vi "chooseParametersFromFiles.vi"(0 "Game in":refnum<class "Game.lvclass">, 1 "AI Parameters":T5={"Defensive Marker"=enum."SecondMostDangerous", "TimeoutDistanceInX"=600.0, "TimeoutDistanceInY"=600.0, "DistanceForaStillBall"=0.0, "TouchDistance"=110.0, "AttackerFarback"=1500.0, "MinDistToKick"=200.0, "Type of Marker"=enum."BlockEnemyPass", "Type of Defense "=enum."Manmark", "PassAngle"=0.045, "KickRange"=60.0, "KickForce"=50.0, "KickEps"=0.05, "KickAngle"=1.0, "Force++"=1.5, "DistanceToKickingAngle"=150.0, "DistanceToBallOut"=600.0, "DistanceStop"=750.0, "DistanceBehindAttacker"=200.0, "Area"=enum."Square", "DistanceForPossession"=180.0, "DistanceToConsirerRobotArrive"=50.0, "DistanceToGoAroundBall"=60.0, "DistanceInFrontOfAttacker"=200.0, "TimeoutDistanceBetweenRobots"=300.0, "MaxOutputAngle"=3.0, "MaxOutputXY"=3.5, "MaxDeceleration"=1.0, "MaxControlIncrement"=1.0, "MaxAcceleration"=4.0, "AngularToleranceForPossession"=0.3, "MaxVelBallToBeginDuelist"=0.5, "ZigZagAngle"=0.0, "PID gains Vel"={"(Kc)"=0.1, "(Ti, min)"=0.0, "(Td, min)"=2.0}, "Number of Offensive"=enum."Auto", "Shoot Out?"=FALSE, "DefenseAvoidArea"=FALSE, "InvertKick"=[], "Simple Pass"=FALSE, "ShootOutForce"=15.0, "dtPosEstBall"=0.3, "AttkIgnoreBallObst"=0.0, "BarrierDist"=130.0, "PassReceiver"=enum."Auto", "GoalieInFrontGoal"=90.0, "RollToPass"=FALSE, "PassReceiver"=enum."Auto", "OldRRT"=FALSE, "Dribbler"=TRUE, "VelNearBall"=2.0, "ChipKick Force"=15.0, "ForcePass\nInGame"=10.0, "bangBangParameters"={"MaxVSent"=2.6, "MaxVNorm"=2.0, "MaxVAng"=6.0, "VAngCircle"=2.5, "LBeginCircle"=300.0, "DistToDestOrientation"=400.0, "MaxVAngToTurn"=6.0, "AtkDistToDestOrientation"=4000.0, "KepperMaxVSent"=3.0, "VelNearEnemy"=1.5}, "BallVelToAbortPass"=1.5, "BallVelToFinishPass"=1.0, "minDistanceToPass"=1000.0, "dribbler_rpm"=1.0, "AttackerAngle\nToTurnInDegrees"=25.0, "AttackerAngle\nToShootInDegrees"=0.5, "distToActivateDibbler"=1000.0, "StopVelocity"=1.2, "timeoutToShoot"=1.5, "DistanceArea"=350.0, "MinDistanceEnemy\nToBallToMark"=750.0, "DisableStopAvoidArea"=FALSE}, 2 "NewParameters":T1={"PenaltyDistance"=0.0, "DistanceAttackerToBackBall"=0.0, "Division"=enum."Div B", "DistanceToAvoidyEnemyRobot"=0.0, "BallPlacementDistance"=900.0, "DisatanceBehindBallToStealBall"=0.0, "MaxDistanceToPositionKickoff"=2000.0, "BlockEnemyTarget"=FALSE, "MaxStopVAng"=1.0, "DistanceMarkerToEnemy"=0.0, "IgnoreDribblerContact"=FALSE, "DistanceToBeginEnemyPosession"=200.0, "GoToBallWhenEnemyNotMoving"=TRUE, "EnemyDistanceToReduceVelocity"=500.0, "TurnOnEnemyDistanceToReduceVelocity"=TRUE, "EnemyDistanceToShootOutBall"=500.0, "DefenseKickBall"=TRUE, "MoreKickToGoal? (0-0.3)"=0.0, "ChipKickInEnemyField"=TRUE, "ShootOutRobotId"=0.0, "FieldLenghtDenominatorInShootOut"=0.0, "AdjustPositionInBallPlacement"=FALSE, "PowerGodPass"=0.0, "VelocityAbortEnemyPos"=0.0, "MaxDistToBeginPass"=500.0, "MinDistToBeginPass"=150.0, "VelocityInDirects"=0.3, "BadDribblerIDs"=[], "NewKickToDistanceAroundBall"=300.0, "PowerAvoidColisionMarker"=0.5, "DistanceToAvoidColisionMarker"=250.0, "AvoidBallKick"=0.0, "DistanceTryKick"=0.0, "SuicideKickDIstance"=0.0, "FirstKickAtck"=FALSE, "AdjustFirstKickDistance"=0.0, "FirstKickDefense"=FALSE, "AvoidAimLessKick"=0.0, "DistanceToAvoidyEnemyShootRobot "=0.0, "NumberOfMarkers"=3.0, "PotField"=TRUE, "PIDLateral"=FALSE, "MinDistanceFirstKickX"=0.0, "MinDistanceFirstKickY"=0.0, "FractionOfDistToTouchGround\nAfterChipKick"=0.8, "FractionOfKickxWhen\nComposedWithKickz"=0.0}, 3 "MainGameConfigs":T2={"SSL UDP RX"={"Local IP:"="", "Server IP:"="224.5.23.2", "Port"="10020"}, "RefBox UDP RX"={"Local IP:"="", "Server IP:"="224.5.23.1", "Port"="10003"}, "Com UDP"={"UDP GrSim TX"=TRUE, "Address:"="172.29.47.23", "Port:"=10301}, "Command"="Force Start", "Goalie"="0", "Side"=enum."Esquerdo", "Team"=enum."Azul"}, 5 "error in (no error)":errorcluster, 7 "ParametersFromFile":T9) -> (14 "Game out":refnum<class "Game.lvclass">, 15 "AI Parameters out":T5={"Defensive Marker"=enum."SecondMostDangerous", "TimeoutDistanceInX"=600.0, "TimeoutDistanceInY"=600.0, "DistanceForaStillBall"=0.0, "TouchDistance"=115.0, "AttackerFarback"=1500.0, "MinDistToKick"=115.0, "Type of Marker"=enum."BlockEnemyPass", "Type of Defense "=enum."Manmark", "PassAngle"=0.045, "KickRange"=60.0, "KickForce"=60.0, "KickEps"=0.05, "KickAngle"=0.09, "Force++"=11.0, "DistanceToKickingAngle"=150.0, "DistanceToBallOut"=600.0, "DistanceStop"=600.0, "DistanceBehindAttacker"=200.0, "Area"=enum."Square", "DistanceForPossession"=180.0, "DistanceToConsirerRobotArrive"=0.0, "DistanceToGoAroundBall"=200.0, "DistanceInFrontOfAttacker"=200.0, "TimeoutDistanceBetweenRobots"=300.0, "MaxOutputAngle"=3.0, "MaxOutputXY"=3.5, "MaxDeceleration"=1.0, "MaxControlIncrement"=1.0, "MaxAcceleration"=4.0, "AngularToleranceForPossession"=0.3, "MaxVelBallToBeginDuelist"=0.5, "ZigZagAngle"=0.0, "PID gains Vel"={"(Kc)"=0.1, "(Ti, min)"=0.0, "(Td, min)"=2.0}, "Number of Offensive"=enum."Auto", "Shoot Out?"=FALSE, "DefenseAvoidArea"=FALSE, "InvertKick"=[], "Simple Pass"=FALSE, "ShootOutForce"=15.0, "dtPosEstBall"=0.3, "AttkIgnoreBallObst"=3000.0, "BarrierDist"=115.0, "PassReceiver"=enum."Auto", "GoalieInFrontGoal"=150.0, "RollToPass"=FALSE, "PassReceiver"=enum."Auto", "OldRRT"=FALSE, "Dribbler"=TRUE, "VelNearBall"=2.0, "ChipKick Force"=2.5, "ForcePass\nInGame"=10.0, "bangBangParameters"={"MaxVSent"=6.5, "MaxVNorm"=1.0, "MaxVAng"=3.0, "VAngCircle"=2.5, "LBeginCircle"=300.0, "DistToDestOrientation"=1000.0, "MaxVAngToTurn"=5.0, "AtkDistToDestOrientation"=4000.0, "KepperMaxVSent"=6.5, "VelNearEnemy"=1.5}, "BallVelToAbortPass"=0.5, "BallVelToFinishPass"=1.0, "minDistanceToPass"=1000.0, "dribbler_rpm"=1000.0, "AttackerAngle\nToTurnInDegrees"=25.0, "AttackerAngle\nToShootInDegrees"=4.0, "distToActivateDibbler"=1000.0, "StopVelocity"=3.5, "timeoutToShoot"=0.0, "DistanceArea"=200.0, "MinDistanceEnemy\nToBallToMark"=800.0, "DisableStopAvoidArea"=FALSE}, 16 "NewParameters out":T1={"PenaltyDistance"=0.0, "DistanceAttackerToBackBall"=0.0, "Division"=enum."Div B", "DistanceToAvoidyEnemyRobot"=0.0, "BallPlacementDistance"=900.0, "DisatanceBehindBallToStealBall"=0.0, "MaxDistanceToPositionKickoff"=2000.0, "BlockEnemyTarget"=FALSE, "MaxStopVAng"=1.0, "DistanceMarkerToEnemy"=0.0, "IgnoreDribblerContact"=FALSE, "DistanceToBeginEnemyPosession"=200.0, "GoToBallWhenEnemyNotMoving"=TRUE, "EnemyDistanceToReduceVelocity"=500.0, "TurnOnEnemyDistanceToReduceVelocity"=TRUE, "EnemyDistanceToShootOutBall"=500.0, "DefenseKickBall"=TRUE, "MoreKickToGoal? (0-0.3)"=0.0, "ChipKickInEnemyField"=TRUE, "ShootOutRobotId"=0.0, "FieldLenghtDenominatorInShootOut"=0.0, "AdjustPositionInBallPlacement"=FALSE, "PowerGodPass"=0.0, "VelocityAbortEnemyPos"=0.0, "MaxDistToBeginPass"=500.0, "MinDistToBeginPass"=150.0, "VelocityInDirects"=0.3, "BadDribblerIDs"=[], "NewKickToDistanceAroundBall"=300.0, "PowerAvoidColisionMarker"=0.5, "DistanceToAvoidColisionMarker"=250.0, "AvoidBallKick"=0.0, "DistanceTryKick"=0.0, "SuicideKickDIstance"=0.0, "FirstKickAtck"=FALSE, "AdjustFirstKickDistance"=0.0, "FirstKickDefense"=FALSE, "AvoidAimLessKick"=0.0, "DistanceToAvoidyEnemyShootRobot "=0.0, "NumberOfMarkers"=3.0, "PotField"=TRUE, "PIDLateral"=FALSE, "MinDistanceFirstKickX"=0.0, "MinDistanceFirstKickY"=0.0, "FractionOfDistToTouchGround\nAfterChipKick"=0.8, "FractionOfKickxWhen\nComposedWithKickz"=0.0}, 17 "MainGameConfigs out":T2={"SSL UDP RX"={"Local IP:"="", "Server IP:"="224.5.23.2", "Port"="10020"}, "RefBox UDP RX"={"Local IP:"="", "Server IP:"="224.5.23.1", "Port"="10003"}, "Com UDP"={"UDP GrSim TX"=TRUE, "Address:"="172.29.47.23", "Port:"=10301}, "Command"="Force Start", "Goalie"="0", "Side"=enum."Esquerdo", "Team"=enum."Azul"}, 19 "error out":errorcluster)   [LabVIEW 2020, in "Game.lvclass"]
uses:
  Game.lvclass
  Controls/PhoenixParameters.ctl
  Play_class/PassReceiver.ctl
  Parameters_class/ChoosePassReceiver.ctl
  Navigation/Controls/bangBangControlParameters.ctl
  MainGameConfigs.ctl
  Controls/vision_control.ctl
  Controls/ComUDP.ctl
  ParametersFromFile.ctl
  Controls/NewParameters.ctl
  Utilities_class/Utilities.lvclass
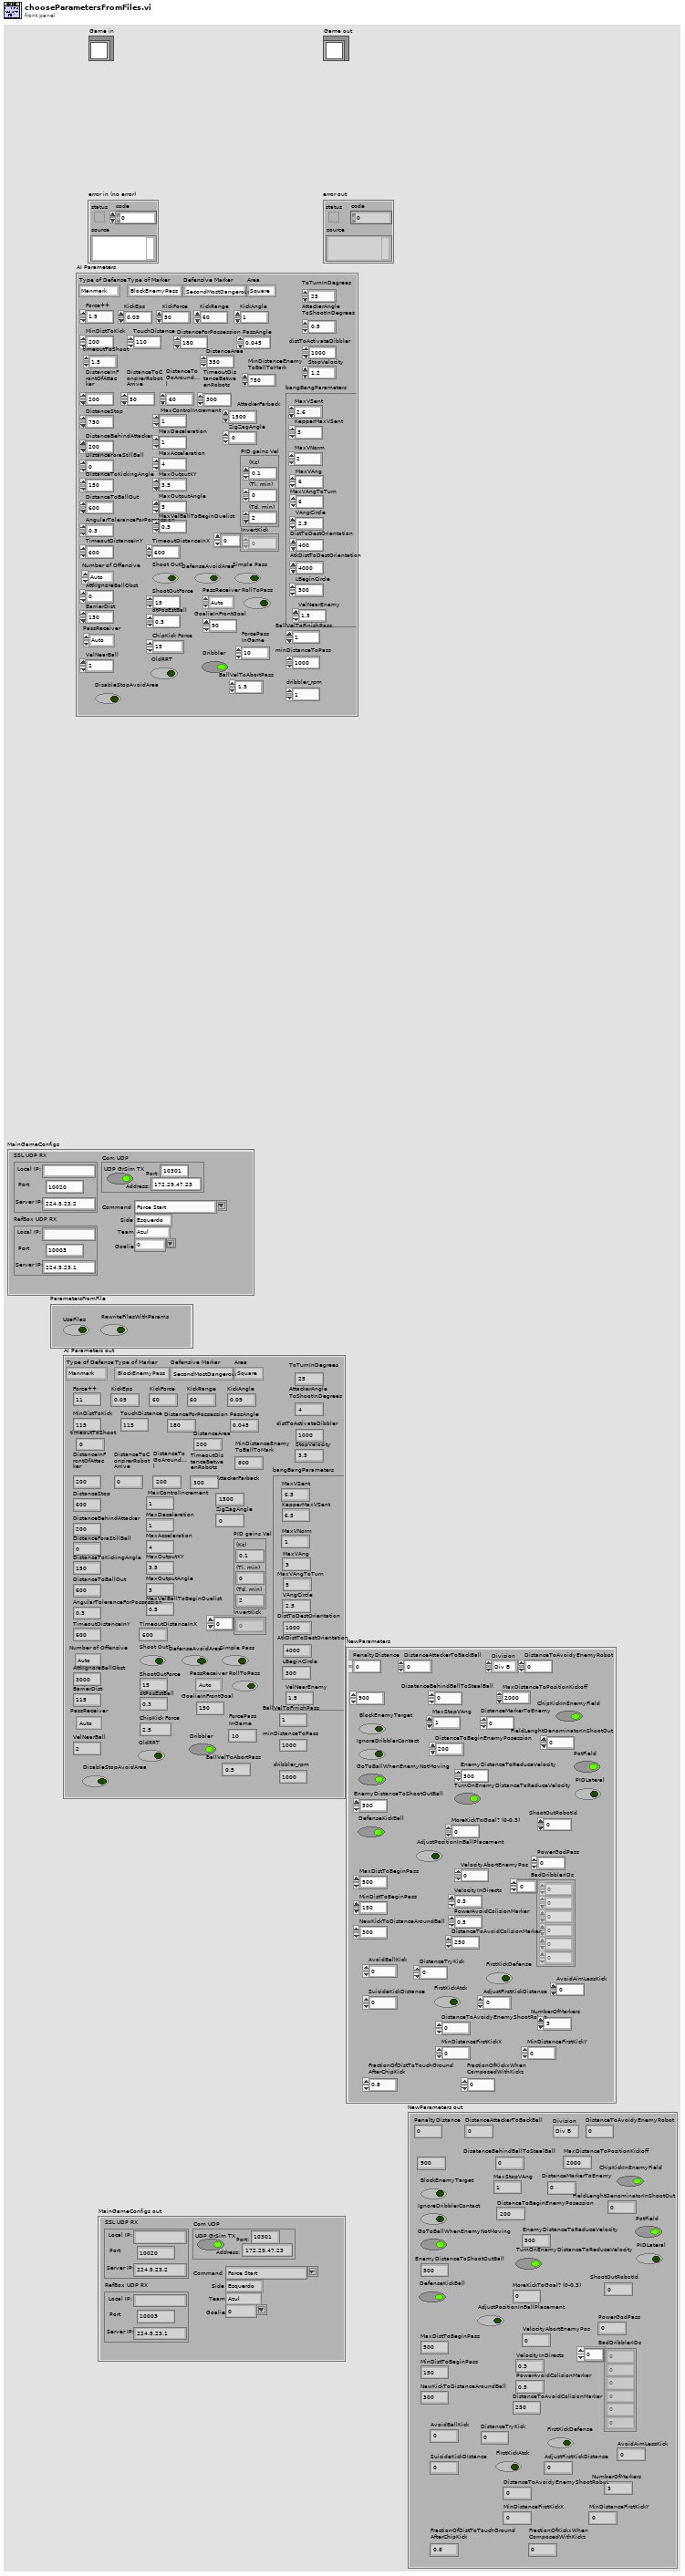
[diagram p1: front panel]
types:
  T1 = typedef "NewParameters.ctl" = cluster{"PenaltyDistance":dbl, "DistanceAttackerToBackBall":dbl, "Division":enum16{"Div B", "Div A"}, "DistanceToAvoidyEnemyRobot":dbl, "BallPlacementDistance":dbl, "DisatanceBehindBallToStealBall":dbl, "MaxDistanceToPositionKickoff":dbl, "BlockEnemyTarget":bool, "MaxStopVAng":dbl, "DistanceMarkerToEnemy":dbl, "IgnoreDribblerContact":bool, "DistanceToBeginEnemyPosession":dbl, "GoToBallWhenEnemyNotMoving":bool, "EnemyDistanceToReduceVelocity":dbl, "TurnOnEnemyDistanceToReduceVelocity":bool, "EnemyDistanceToShootOutBall":dbl, "DefenseKickBall":bool, "MoreKickToGoal? (0-0.3)":dbl, "ChipKickInEnemyField":bool, "ShootOutRobotId":dbl, "FieldLenghtDenominatorInShootOut":dbl, "AdjustPositionInBallPlacement":bool, "PowerGodPass":dbl, "VelocityAbortEnemyPos":dbl, "MaxDistToBeginPass":dbl, "MinDistToBeginPass":dbl, "VelocityInDirects":dbl, "BadDribblerIDs":i32[], "NewKickToDistanceAroundBall":dbl, "PowerAvoidColisionMarker":dbl, "DistanceToAvoidColisionMarker":dbl, "AvoidBallKick":dbl, "DistanceTryKick":dbl, "SuicideKickDIstance":dbl, "FirstKickAtck":bool, "AdjustFirstKickDistance":dbl, "FirstKickDefense":bool, "AvoidAimLessKick":dbl, "DistanceToAvoidyEnemyShootRobot ":dbl, "NumberOfMarkers":dbl, "PotField":bool, "PIDLateral":bool, "MinDistanceFirstKickX":dbl, "MinDistanceFirstKickY":dbl, "FractionOfDistToTouchGround\nAfterChipKick":dbl, "FractionOfKickxWhen\nComposedWithKickz":dbl}
  T2 = typedef "MainGameConfigs.ctl" = cluster{"SSL UDP RX":T3, "RefBox UDP RX":T3, "Com UDP":T4, "Command":string, "Goalie":string, "Side":enum16{"Esquerdo", "Direito"}, "Team":enum16{"Azul", "Amarelo"}}
  T3 = typedef "vision_control.ctl" = cluster{"Local IP:":string, "Server IP:":string, "Port":string}
  T4 = typedef "ComUDP.ctl" = cluster{"UDP GrSim TX":bool, "Address:":string, "Port:":u16}
  T5 = typedef "PhoenixParameters.ctl" = cluster{"Defensive Marker":enum16{"SecondMostDangerous", "MostDangerous"}, "TimeoutDistanceInX":dbl, "TimeoutDistanceInY":dbl, "DistanceForaStillBall":dbl, "TouchDistance":dbl, "AttackerFarback":dbl, "MinDistToKick":dbl, "Type of Marker":enum16{"BlockEnemyPass", "BlockOurGoal"}, "Type of Defense ":enum16{"Barreira", "Manmark"}, "PassAngle":dbl, "KickRange":dbl, "KickForce":dbl, "KickEps":dbl, "KickAngle":dbl, "Force++":dbl, "DistanceToKickingAngle":dbl, "DistanceToBallOut":dbl, "DistanceStop":dbl, "DistanceBehindAttacker":dbl, "Area":enum16{"Circular", "Square"}, "DistanceForPossession":dbl, "DistanceToConsirerRobotArrive":dbl, "DistanceToGoAroundBall":dbl, "DistanceInFrontOfAttacker":dbl, "TimeoutDistanceBetweenRobots":dbl, "MaxOutputAngle":dbl, "MaxOutputXY":dbl, "MaxDeceleration":dbl, "MaxControlIncrement":dbl, "MaxAcceleration":dbl, "AngularToleranceForPossession":dbl, "MaxVelBallToBeginDuelist":dbl, "ZigZagAngle":dbl, "PID gains Vel":cluster{"(Kc)":dbl, "(Ti, min)":dbl, "(Td, min)":dbl}, "Number of Offensive":enum16{"6", "5", "4", "3", "2", "1", "0", "Auto"}, "Shoot Out?":bool, "DefenseAvoidArea":bool, "InvertKick":dbl[], "Simple Pass":bool, "ShootOutForce":dbl, "dtPosEstBall":dbl, "AttkIgnoreBallObst":dbl, "BarrierDist":dbl, "PassReceiver":T6, "GoalieInFrontGoal":dbl, "RollToPass":bool, "PassReceiver":T7, "OldRRT":bool, "Dribbler":bool, "VelNearBall":dbl, "ChipKick Force":dbl, "ForcePass\nInGame":dbl, "bangBangParameters":T8, "BallVelToAbortPass":dbl, "BallVelToFinishPass":dbl, "minDistanceToPass":dbl, "dribbler_rpm":dbl, "AttackerAngle\nToTurnInDegrees":dbl, "AttackerAngle\nToShootInDegrees":dbl, "distToActivateDibbler":dbl, "StopVelocity":dbl, "timeoutToShoot":dbl, "DistanceArea":dbl, "MinDistanceEnemy\nToBallToMark":dbl, "DisableStopAvoidArea":bool}
  T6 = typedef "PassReceiver.ctl" = enum16{"Auto", "2ndStriker", "Striker"}
  T7 = typedef "ChoosePassReceiver.ctl" = enum16{"Striker", "2ndStriker", "Auto"}
  T8 = typedef "bangBangControlParameters.ctl" = cluster{"MaxVSent":dbl, "MaxVNorm":dbl, "MaxVAng":dbl, "VAngCircle":dbl, "LBeginCircle":dbl, "DistToDestOrientation":dbl, "MaxVAngToTurn":dbl, "AtkDistToDestOrientation":dbl, "KepperMaxVSent":dbl, "VelNearEnemy":dbl}
  T9 = typedef "ParametersFromFile.ctl" = cluster{"UseFiles":bool, "RewriteFilesWithParams":bool}
  T10 = enum16{"open", "replace", "create", "open or create", "replace or create", "replace or create with confirmation"}
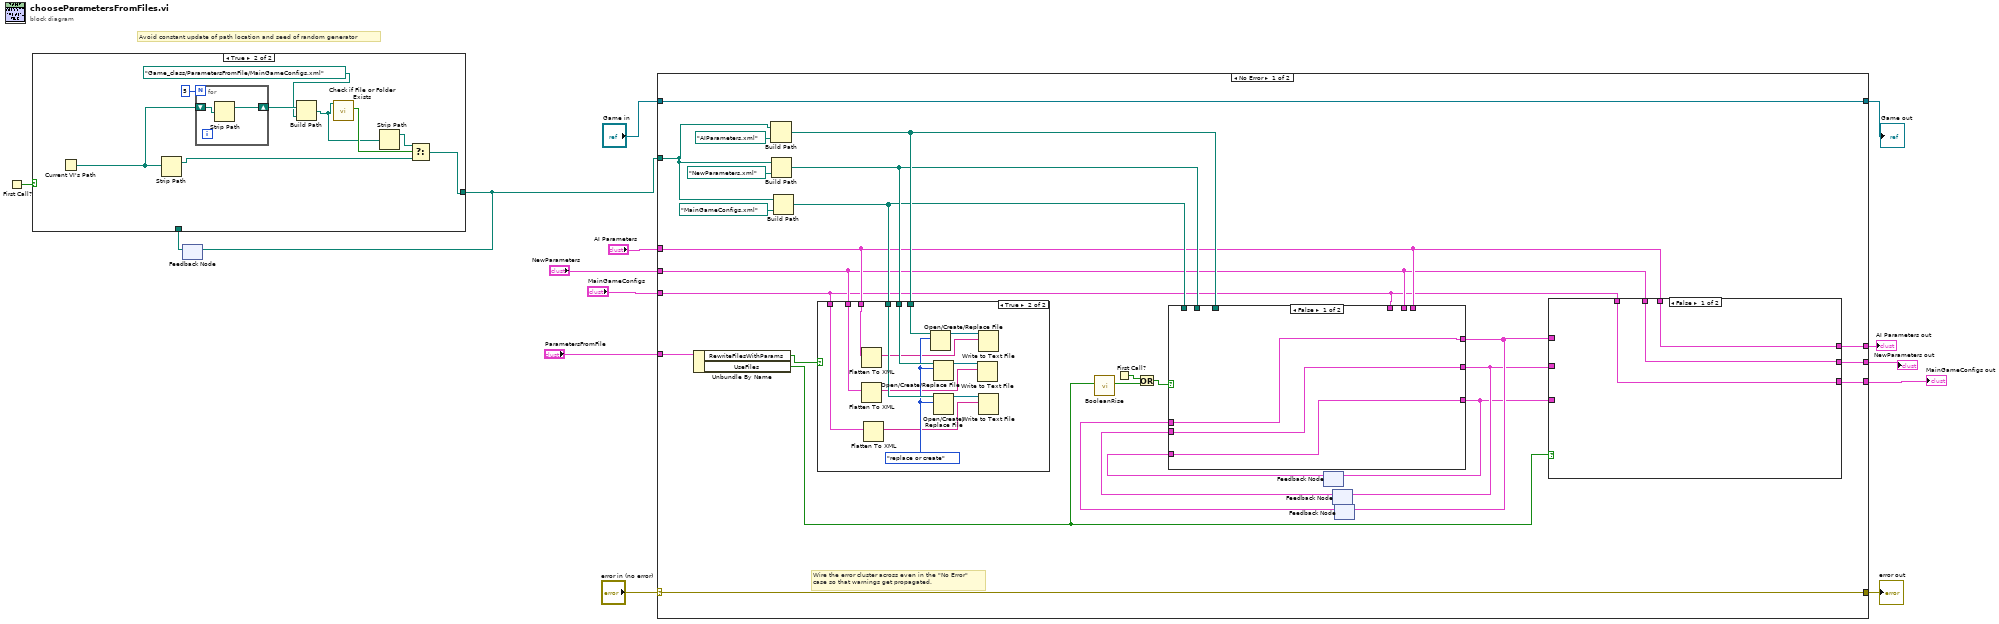
[diagram p0: block diagram]
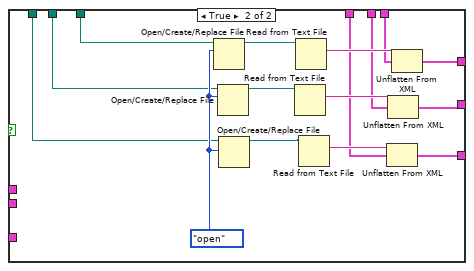
[diagram p3: hidden frame]
diagram:
  # "Avoid constant update of path location and seed of random generator"
  n1 = First Call?() -> (First Call?: T/F=w3:bool)
  n2 = feedback #1() -> (w7:path)  [unwired: 1 in]
  n3 = case shown="True" w3 {
    tunnel: [w15 w21] -> w6
    tunnel: w7 -> [w15 _]
    frame False {
    }
    frame True {
      n4 = Current VI's Path() -> (path=w16:path)
      n5 = Strip Path(path=w16) -> (stripped path=w19:path)  [unwired: 1 out]
      n6 = for {
        N: 5 -> [_]
        shift-right: [w25] -> w23
        shift-left: w16 -> [w26]
        n7 = Strip Path(path=w26) -> (stripped path=w25:path)  [unwired: 1 out]
      }
      n8 = Build Path(base path=w23, name or relative path=path "Game_class/ParametersFromFile/MainGameConfigs.xml") -> (appended path=w18:path)
      n9 = call <vilib>:"Check if File or Folder Exists.vi"("path"=w18) -> ("file or folder exists?"=w20:bool)  [unwired: 8 in, 2 out]
      n10 = Strip Path(path=w18) -> (stripped path=w17:path)  [unwired: 1 out]
      n11 = Select(t=w17, s=w20, f=w19) -> (s? t:f=w21:path)
    }
  }
  n12 = feedback-in #1(w6) -> ()
  n13 = case shown="No Error" "error in (no error)" {
    selector: "error in (no error)" -> [w52 w93]
    tunnel: [w52 w93] -> w13
    tunnel: [w53 w92] -> w11
    tunnel: "Game in" -> [w53 w92]
    tunnel: "AI Parameters" -> [w41 _]
    tunnel: "NewParameters" -> [w40 _]
    tunnel: "MainGameConfigs" -> [w39 _]
    tunnel: "ParametersFromFile" -> [w47 _]
    tunnel: w6 -> [w48 _]
    tunnel: [w32 _] -> w5
    tunnel: [w31 _] -> w1
    tunnel: [w30 _] -> w4
    frame No Error {
      # "Wire the error cluster across even in the \"No Error\"\ncase so that warnings get propagated."
      n14 = Unbundle By Name(w47) -> ("RewriteFilesWithParams"=w46:bool, "UseFiles"=w45:bool)
      n15 = Build Path(base path=w48, name or relative path=path "AIParameters.xml") -> (appended path=w44:path)
      n16 = Build Path(base path=w48, name or relative path=path "NewParameters.xml") -> (appended path=w43:path)
      n17 = Build Path(base path=w48, name or relative path=path "MainGameConfigs.xml") -> (appended path=w42:path)
      n18 = case shown="True" w46 {
        tunnel: w41 -> [_ w84]
        tunnel: w40 -> [_ w82]
        tunnel: w39 -> [_ w80]
        tunnel: w44 -> [_ w91]
        tunnel: w43 -> [_ w90]
        tunnel: w42 -> [_ w89]
        frame False {
        }
        frame True {
          w88 = T10."replace or create" ("operation (0:open)")
          n19 = Flatten To XML(6:w84) -> (2:w83:string)
          n20 = Flatten To XML(6:w82) -> (2:w81:string)
          n21 = Flatten To XML(6:w80) -> (2:w79:string)
          n22 = Open/Create/Replace File(file path (use dialog)=w91, operation (0:open)=w88) -> (refnum out=w87:refnum<file>)  [unwired: 4 in, 2 out]
          n23 = Open/Create/Replace File(file path (use dialog)=w90, operation (0:open)=w88) -> (refnum out=w86:refnum<file>)  [unwired: 4 in, 2 out]
          n24 = Open/Create/Replace File(file path (use dialog)=w89, operation (0:open)=w88) -> (refnum out=w85:refnum<file>)  [unwired: 4 in, 2 out]
          n25 = Write to Text File(file (use dialog)=w86, text=w81) -> ()  [unwired: 2 in, 3 out]
          n26 = Write to Text File(file (use dialog)=w87, text=w83) -> ()  [unwired: 2 in, 3 out]
          n27 = Write to Text File(file (use dialog)=w85, text=w79) -> ()  [unwired: 2 in, 3 out]
        }
      }
      n28 = call "BooleanRise.vi"("Boolean in"=w45) -> ("Boolean"=w28:bool)  [unwired: 8 in, 2 out]
      n29 = First Call?() -> (First Call?: T/F=w29:bool)
      n30 = Or(x=w29, y=w28) -> (x .or. y?=w27:bool)
      n31 = feedback #2() -> (w38:T2)  [unwired: 1 in]
      n32 = feedback #3() -> (w37:T1)  [unwired: 1 in]
      n33 = feedback #4() -> (w36:T5)  [unwired: 1 in]
      n34 = case shown="False" w27 {
        tunnel: w44 -> [_ w68]
        tunnel: w43 -> [_ w67]
        tunnel: w42 -> [_ w66]
        tunnel: w41 -> [_ w62]
        tunnel: w40 -> [_ w61]
        tunnel: w39 -> [_ w60]
        tunnel: [w56 w59] -> w35
        tunnel: [w55 w58] -> w34
        tunnel: [w54 w57] -> w33
        tunnel: w38 -> [w54 _]
        tunnel: w37 -> [w55 _]
        tunnel: w36 -> [w56 _]
        frame False {
        }
        frame True {
          w69 = T10."open" ("operation (0:open)")
          n35 = Open/Create/Replace File(file path (use dialog)=w68, operation (0:open)=w69) -> (refnum out=w72:refnum<file>)  [unwired: 4 in, 2 out]
          n36 = Open/Create/Replace File(file path (use dialog)=w67, operation (0:open)=w69) -> (refnum out=w71:refnum<file>)  [unwired: 4 in, 2 out]
          n37 = Open/Create/Replace File(file path (use dialog)=w66, operation (0:open)=w69) -> (refnum out=w70:refnum<file>)  [unwired: 4 in, 2 out]
          n38 = Read from Text File(file (use dialog)=w71) -> (text=w64:string)  [unwired: 3 in, 3 out]
          n39 = Read from Text File(file (use dialog)=w72) -> (text=w65:string)  [unwired: 3 in, 3 out]
          n40 = Read from Text File(file (use dialog)=w70) -> (text=w63:string)  [unwired: 3 in, 3 out]
          n41 = Unflatten From XML(xml string=w63, type=w60) -> (value=w57:T2)  [unwired: 1 in, 1 out]
          n42 = Unflatten From XML(xml string=w64, type=w61) -> (value=w58:T1)  [unwired: 1 in, 1 out]
          n43 = Unflatten From XML(xml string=w65, type=w62) -> (value=w59:T5)  [unwired: 1 in, 1 out]
        }
      }
      n44 = feedback-in #2(w33) -> ()
      n45 = feedback-in #3(w34) -> ()
      n46 = feedback-in #4(w35) -> ()
      n47 = case shown="False" w45 {
        tunnel: w41 -> [w75 _]
        tunnel: w40 -> [w74 _]
        tunnel: w39 -> [w73 _]
        tunnel: [w75 w78] -> w32
        tunnel: [w74 w77] -> w31
        tunnel: [w73 w76] -> w30
        tunnel: w35 -> [_ w78]
        tunnel: w34 -> [_ w77]
        tunnel: w33 -> [_ w76]
        frame False {
        }
        frame True {
        }
      }
    }
    frame Error {
    }
  }
  "error out" <- w13
  "Game out" <- w11
  "AI Parameters out" <- w5
  "MainGameConfigs out" <- w4
  "NewParameters out" <- w1
